vi "Determine Clothoid Values.vi"(10 "Scaling":dbl, 11 "Desired Length":dbl) -> (0 "Center Point":cluster{dbl, dbl}, 1 "Tangent Angle rad":dbl, 2 "Para Time":dbl, 3 "Vertex Dist ft":dbl, 4 "Radius":dbl)   [LabVIEW 2019]
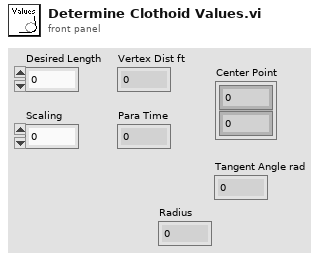
[diagram p1: front panel]
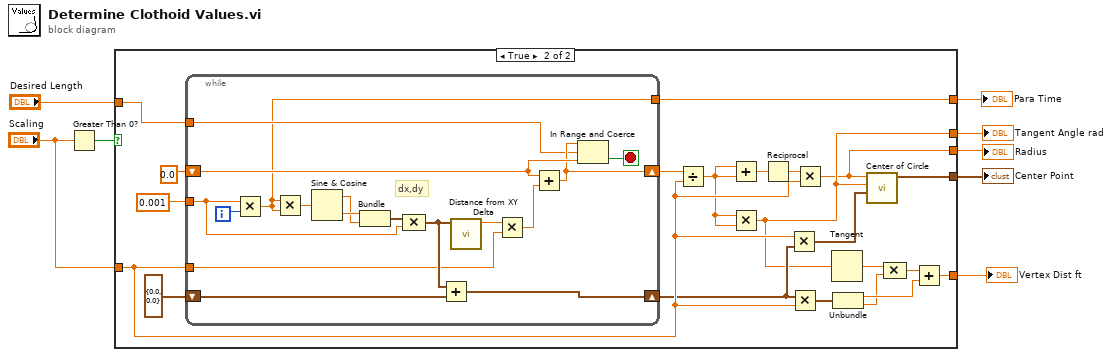
[diagram p0: block diagram]
diagram:
  n1 = Greater Than 0?(x="Scaling") -> (x > 0?=w6:bool)
  n2 = case shown="True" w6 {
    tunnel: "Scaling" -> [_ w14]
    tunnel: [_ w22] -> w8
    tunnel: "Desired Length" -> [_ w20]
    tunnel: [_ w19] -> w4
    tunnel: [_ w15] -> w3
    tunnel: [_ w10] -> w2
    tunnel: [_ w9] -> w1
    frame False {
    }
    frame True {
      n3 = while {
        shift-right: [w36] -> w13
        shift-left: cluster{dbl, dbl} {0.0, 0.0} -> [w41]
        tunnel: 0.001 -> [w40]
        shift-right: [w38] -> w16
        shift-left: 0.0 -> [w39]
        tunnel: w14 -> [w30]
        tunnel: w20 -> [w34]
        tunnel: [w33] -> w19
        i -> [w46]
        stop <- w37 stop-if-true
        # "dx,dy"
        n4 = Multiply(x=w40, y=w46) -> (x*y=w33:dbl)
        n5 = Multiply(x=w33, y=w33) -> (x*y=w45:dbl)
        n6 = Sine & Cosine(0:w45) -> (1:w43:dbl, 2:w44:dbl)
        n7 = Bundle(w44, w43) -> (w42:cluster{dbl, dbl})  [unwired: 1 in]
        n8 = Compound Arithmetic op=MULTIPLY(w42, w40) -> (w32:cluster{dbl, dbl})
        n9 = Add(x=w32, y=w41) -> (x+y=w36:cluster{dbl, dbl})
        n10 = call "Distance from XY Delta.vi"("Delta Point"=w32) -> ("Distance"=w31:dbl)  [unwired: 10 in]
        n11 = Multiply(x=w31, y=w30) -> (x*y=w35:dbl)
        n12 = Add(x=w39, y=w35) -> (x+y=w38:dbl)
        n13 = In Range and Coerce(upper limit=w38, x=w34, lower limit=w39) -> (In Range?=w37:bool)  [unwired: 1 out]
      }
      n14 = Divide(x=w16, y=w14) -> (x/y=w11:dbl)
      n15 = Add(x=w11, y=w11) -> (x+y=w18:dbl)
      n16 = Multiply(x=w11, y=w11) -> (x*y=w10:dbl)
      n17 = Reciprocal(x=w18) -> (1/x=w17:dbl)
      n18 = Multiply(x=w14, y=w13) -> (x*y=w12:cluster{dbl, dbl})
      n19 = Multiply(x=w13, y=w14) -> (x*y=w21:cluster{dbl, dbl})
      n20 = Multiply(x=w17, y=w14) -> (x*y=w9:dbl)
      n21 = Tangent(1:w10) -> (0:w23:dbl)
      n22 = Unbundle(w21) -> (w26:dbl, w24:dbl)
      n23 = call "Center of Circle.vi"("Tangent Point"=w12, "Tangent Angle"=w10, "Radius"=w9) -> ("Center Point"=w15:cluster{dbl, dbl})  [unwired: 8 in]
      n24 = Compound Arithmetic op=MULTIPLY(w23, w24) -> (w25:dbl)
      n25 = Add(x=w25, y=w26) -> (x+y=w22:dbl)
    }
  }
  "Vertex Dist ft" <- w8
  "Para Time" <- w4
  "Center Point" <- w3
  "Tangent Angle rad" <- w2
  "Radius" <- w1
